vi "Write difftrack.vi"(8 "error in (no error)":errorcluster, 10 "Difftrack.lvclass":refnum<class "Difftrack.lvclass">, 11 "Target in":refnum<class "Target.lvclass">) -> (0 "error out":errorcluster, 3 "Target out":refnum<class "Target.lvclass">)   [LabVIEW 2014, in "TCSDataDefinitions.lvlib" / "TCSCommand.lvlib" / "TargetConfiguration.lvlib" / "Target.lvlib" / "Target.lvclass"]
uses:
  Target/Target.lvclass
  Difftrack/Difftrack.lvclass
  Target/Target.lvclass/Target.ctl
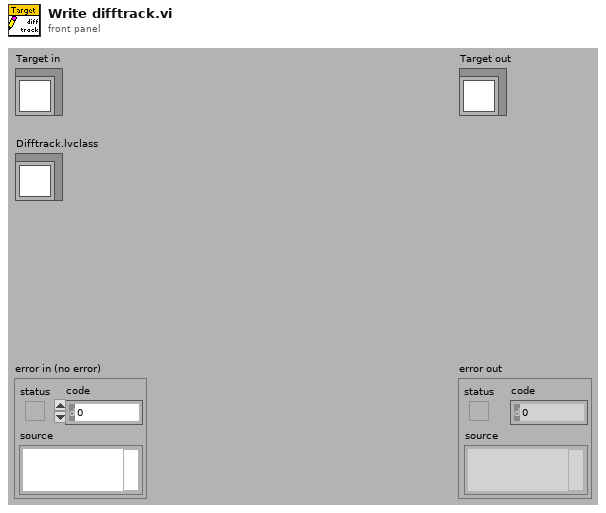
[diagram p1: front panel]
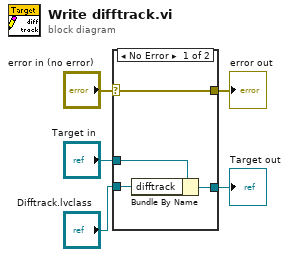
[diagram p0: block diagram]
diagram:
  n1 = case shown="No Error" "error in (no error)" {
    selector: "error in (no error)" -> [w9 w10]
    tunnel: [w9 w10] -> w4
    tunnel: [w7 w11] -> w2
    tunnel: "Target in" -> [w8 w11]
    tunnel: "Difftrack.lvclass" -> [w6 _]
    frame No Error {
      n2 = Bundle By Name(cluster=w8, "difftrack"=w6) -> (w7:refnum<class "Target.lvclass">)
    }
    frame Error {
    }
  }
  "error out" <- w4
  "Target out" <- w2
